vi "NI9482_driver.vi"(6 "MethodNI9482":T1, 8 "error in (no error)":errorcluster, 10 "Data 4 RLY":bool[](array[boolean]), 11 "Line(s)NI9482":tag="Dev1/port0/line0:7") -> (0 "error out":errorcluster, 3 "ok?":bool)   [LabVIEW 2020]
uses:
  TYPEDEF/NI9482_TD_Method.ctl
  <vilib>/DAQmx/write.llb/DAQmx Write (Digital 1D Bool 1Chan 1Samp).vi
  <vilib>/DAQmx/create/channels.llb/DAQmx Create Channel (DO-Digital Output).vi
  <vilib>/DAQmx/miscellaneous.llb/DAQmx Fill In Error Info.vi
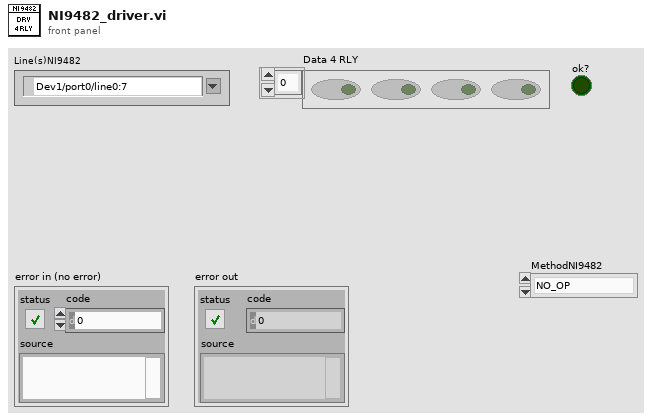
[diagram p1: front panel]
types:
  T1 = typedef "NI9482_TD_Method.ctl" = enum16{"NO_OP", "INIT", "SET", "CLOSE", "END"}
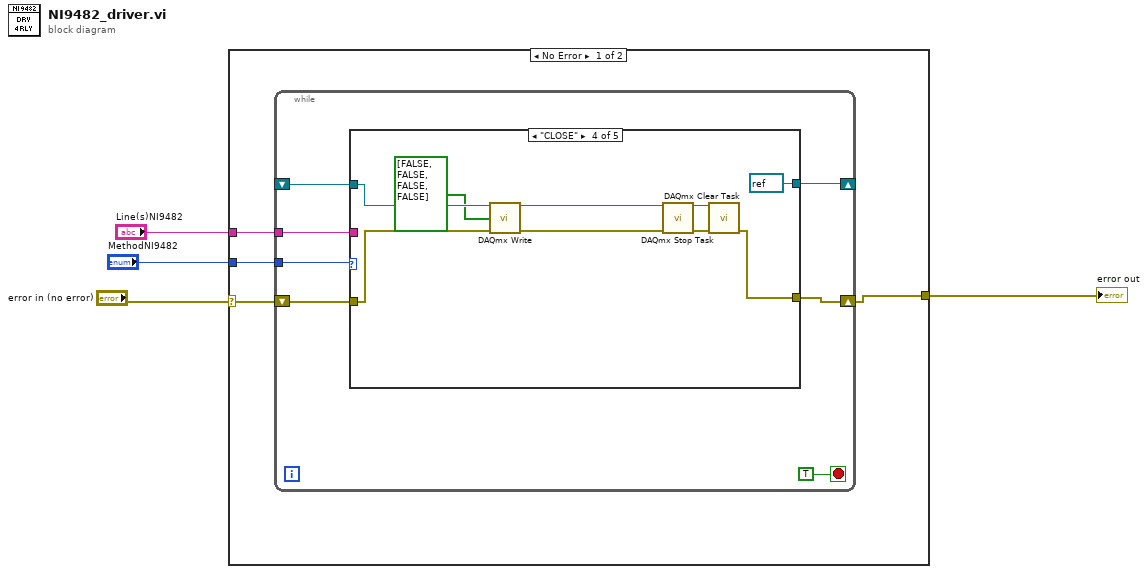
[diagram p0: block diagram]
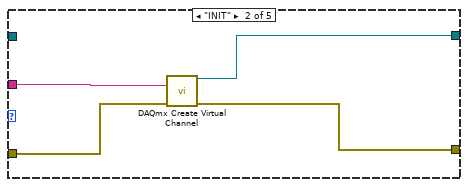
[diagram p3: hidden frame]
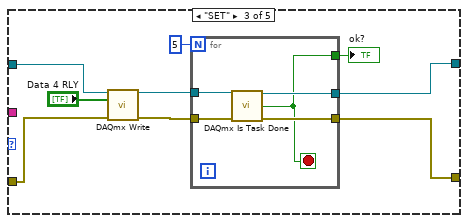
[diagram p4: hidden frame]
diagram:
  n1 = case shown="No Error" "error in (no error)" {
    selector: "error in (no error)" -> [w6 w47]
    tunnel: "MethodNI9482" -> [w8 _]
    tunnel: "Line(s)NI9482" -> [w7 _]
    tunnel: [w5 w47] -> w1
    frame No Error {
      n2 = while {
        tunnel: w8 -> [w14]
        tunnel: w7 -> [w13]
        shift-right: [w11] -> w5
        shift-left: w6 -> [w12]
        shift-right: [w10] -> _
        shift-left: _ -> [w9]
        stop <- TRUE stop-if-true
        n3 = case shown="\"CLOSE\"" w14 {
          tunnel: w13 -> [_ w21 _ _ _]
          tunnel: w12 -> [w16 w20 w29 w38 w45]
          tunnel: [w16 w19 w23 w42 w45] -> w11
          tunnel: [w17 w18 w24 refnum<k21> refnum ("task out") w46] -> w10
          tunnel: w9 -> [w17 _ w28 w41 w46]
          frame "NO_OP", Default {
          }
          frame "INIT" {
            n4 = call-poly <vilib>:"DAQmx Create Virtual Channel.vi"("lines"=w21, "error in"=w20) -> ("task out"=w18:refnum<k21>, "error out"=w19:errorcluster)  [unwired: 12 in]
          }
          frame "SET" {
            n5 = call-poly <vilib>:"DAQmx Write.vi"("task/channels in"=w28, "data"="Data 4 RLY", "error in"=w29) -> ("task out"=w27:refnum<k21>, "error out"=w26:errorcluster)  [unwired: 10 in, 1 out]
            n6 = for {
              N: 5 -> [_]
              tunnel: w27 -> [w35]
              tunnel: w26 -> [w34]
              tunnel: [w33] -> w24
              tunnel: [w32] -> w23
              tunnel: [w31] -> w22
              stop <- w31 stop-if-true
              n7 = call <vilib>:"DAQmx Is Task Done.vi"("task/channels in"=w35, "error in"=w34) -> ("task out"=w33:refnum<k21>, "task done?"=w31:bool, "error out"=w32:errorcluster)  [unwired: 11 in]
            }
            "ok?" <- w22
          }
          frame "CLOSE" {
            n8 = call-poly <vilib>:"DAQmx Write.vi"("task/channels in"=w41, "data"=bool[] [FALSE, FALSE, FALSE, FALSE], "error in"=w38) -> ("task out"=w40:refnum<k21>, "error out"=w39:errorcluster)  [unwired: 10 in, 1 out]
            n9 = call <vilib>:"DAQmx Stop Task.vi"("task/channels in"=w40, "error in"=w39) -> ("task out"=w43:refnum<k21>, "error out"=w44:errorcluster)  [unwired: 12 in]
            n10 = call <vilib>:"DAQmx Clear Task.vi"("task in"=w43, "error in"=w44) -> ("error out"=w42:errorcluster)  [unwired: 13 in]
          }
          frame "END" {
          }
        }
      }
    }
    frame Error {
    }
  }
  "error out" <- w1
